vi "Accelerometer.vi"() -> ()   [LabVIEW 2017]
uses:
  <vilib>/DAQmx/read.llb/DAQmx Read (Analog 1D Wfm NChan NSamp).vi
  <vilib>/DAQmx/miscellaneous.llb/DAQmx Fill In Error Info.vi
panel:
  out "Waveform Chart":cluster{"Waveform":dbl, "Waveform":dbl}[](graph)
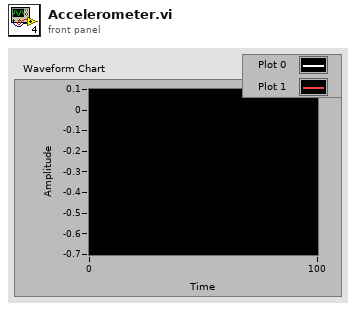
[diagram p1: front panel]
types:
  T1 = cluster{"Waveform":waveform(dbl), "Waveform":waveform(dbl)}[]
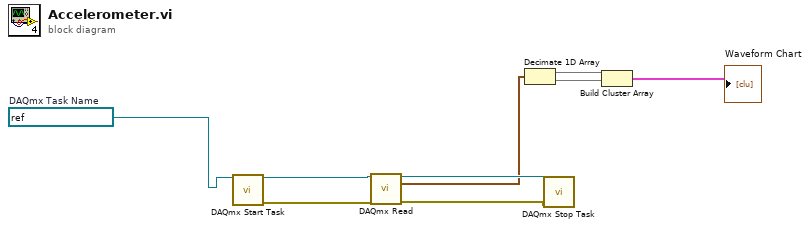
[diagram p0: block diagram]
diagram:
  w7 = refnum<k21> "Accelerometer"  # DAQmx Task Name
  n1 = call <vilib>:"DAQmx Start Task.vi"("task/channels in"=w7) -> ("task out"=w6:refnum<k21>, "error out"=w9:errorcluster)  [unwired: 13 in]
  n2 = call-poly <vilib>:"DAQmx Read.vi"("task/channels in"=w6, "error in"=w9) -> ("task out"=w5:refnum<k21>, "data"=w4:waveform(dbl)[], "error out"=w8:errorcluster)  [unwired: 11 in]
  n3 = Decimate 1D Array(w4) -> (w3:waveform(dbl)[], w2:waveform(dbl)[])
  n4 = call <vilib>:"DAQmx Stop Task.vi"("task/channels in"=w5, "error in"=w8) -> ()  [unwired: 12 in, 2 out]
  n5 = Build Cluster Array(w3, w2) -> (→"Waveform Chart":T1)
